vi "Sample Power-DAQ-Stats_custom.vi"() -> ()   [LabVIEW 2018]
panel:
  in  "file path":path=path "C:/Users/aspit/OneDrive/Data/TRMC/Power Meter"
  out "Power Value":sgl=6.999518e-05 format="%^#_6g"
  in  "milliseconds to wait":u32
  in  "stop":bool
  out "Device Key length":i32=14
  out "Device Key":string="1936-R SN46426"
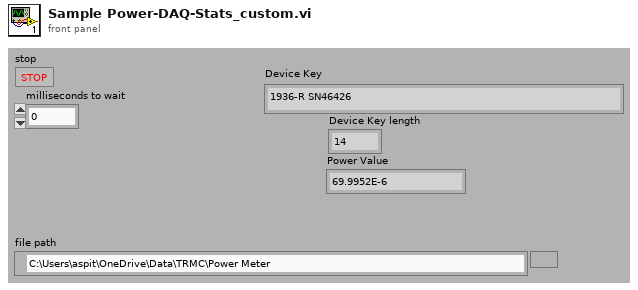
[diagram p1: front panel]
types:
  T1 = enum16{"open", "open or create", "create or replace", "create", "open (read-only)"}
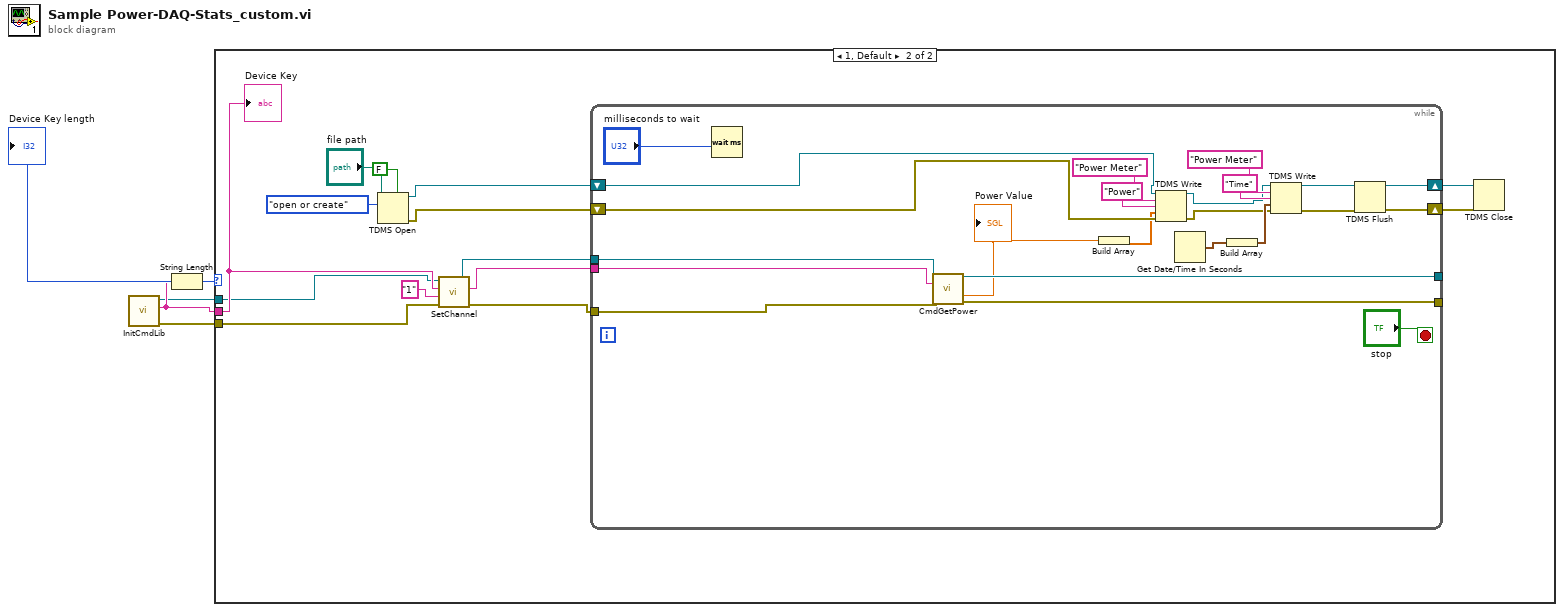
[diagram p0: block diagram]
diagram:
  n1 = call "InitCmdLib.vi"() -> ("error out"=w2:errorcluster, "Device Key"=w3:string, "CmdLib"=w1:refnum<k24>)  [unwired: 9 in]
  n2 = String Length(string=w3) -> (length=w4:i32)
  "Device Key length" <- w4
  n3 = case shown="1, Default" w4 {
    tunnel: w3 -> [_ w18]
    tunnel: w2 -> [_ w17]
    tunnel: w1 -> [_ w15]
    frame 0 {
    }
    frame 1, Default {
      n4 = TDMS Open(5:FALSE ("create index file? (T)"), 10:T1."open or create" ("operation (0:open)"), 11:"file path") -> (0:w7:errorcluster, 3:w8:refnum<k34>)  [unwired: 4 in]
      n5 = call "SetChannel.vi"("error in"=w17, "Channel 1 or 2"="1" ("channel"), "Device Key In"=w18, "PM Cmds In"=w15) -> ("error out"=w14:errorcluster, "Device Key Out"=w13:string, "PM Cmds Out"=w12:refnum<k24>)  [unwired: 1 in]
      n6 = while {
        tunnel: [w41] -> _
        tunnel: [w40] -> _
        tunnel: w14 -> [w37]
        tunnel: w13 -> [w36]
        tunnel: w12 -> [w35]
        shift-right: [w20] -> w6
        shift-left: w8 -> [w34]
        shift-right: [w19] -> w5
        shift-left: w7 -> [w33]
        stop <- "stop" stop-if-true
        n7 = Wait (ms)(milliseconds to wait="milliseconds to wait") -> ()  [unwired: 1 out]
        n8 = call "CmdGetPower.vi"("PM Cmds In"=w35, "Device Key In"=w36, "error in"=w37) -> ("PM Cmds Out"=w41:refnum<k24>, "Power Value"=w31:sgl, "error out"=w40:errorcluster)  [unwired: 8 in, 2 out]
        "Power Value" <- w31
        n9 = Build Array(w31) -> (w30:sgl[])
        n10 = TDMS Write(0:w34, 5:"Power Meter" ("group name in (Untitled)"), 7:"Power" ("group name in (Untitled)"), 9:w30, 11:w33) -> (4:w24:refnum<k34>, 15:w23:errorcluster)  [unwired: 1 in, 2 out]
        n11 = Get Date/Time In Seconds() -> (seconds since 1Jan1904=w26:timestamp)
        n12 = Build Array(w26) -> (w25:timestamp[])
        n13 = TDMS Write(0:w24, 5:"Power Meter" ("group name in (Untitled)"), 7:"Time" ("group name in (Untitled)"), 9:w25, 11:w23) -> (4:w22:refnum<k34>, 15:w21:errorcluster)  [unwired: 1 in, 2 out]
        n14 = TDMS Flush(4:w21, 7:w22) -> (0:w19:errorcluster, 3:w20:refnum<k34>)
      }
      n15 = TDMS Close(8:w5, 11:w6) -> ()  [unwired: 2 out]
      "Device Key" <- w18
    }
  }
